vi "VA_ExtractImg32.vi"(1 "y":sgl, 2 "x":sgl, 3 "Image Src":T1) -> (0 "Image Dst Out":T1)   [LabVIEW 2009]
uses:
  <vilib>/vision/Image Controls.llb/IMAQ Image.ctl
  <vilib>/vision/NI_Vision_Development_Module.lvlib
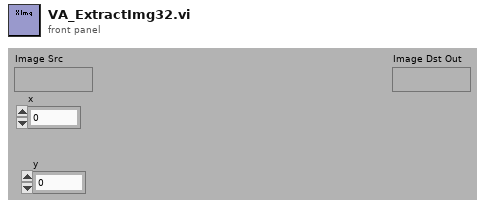
[diagram p1: front panel]
types:
  T1 = typedef "IMAQ Image.ctl" = refnum<image>
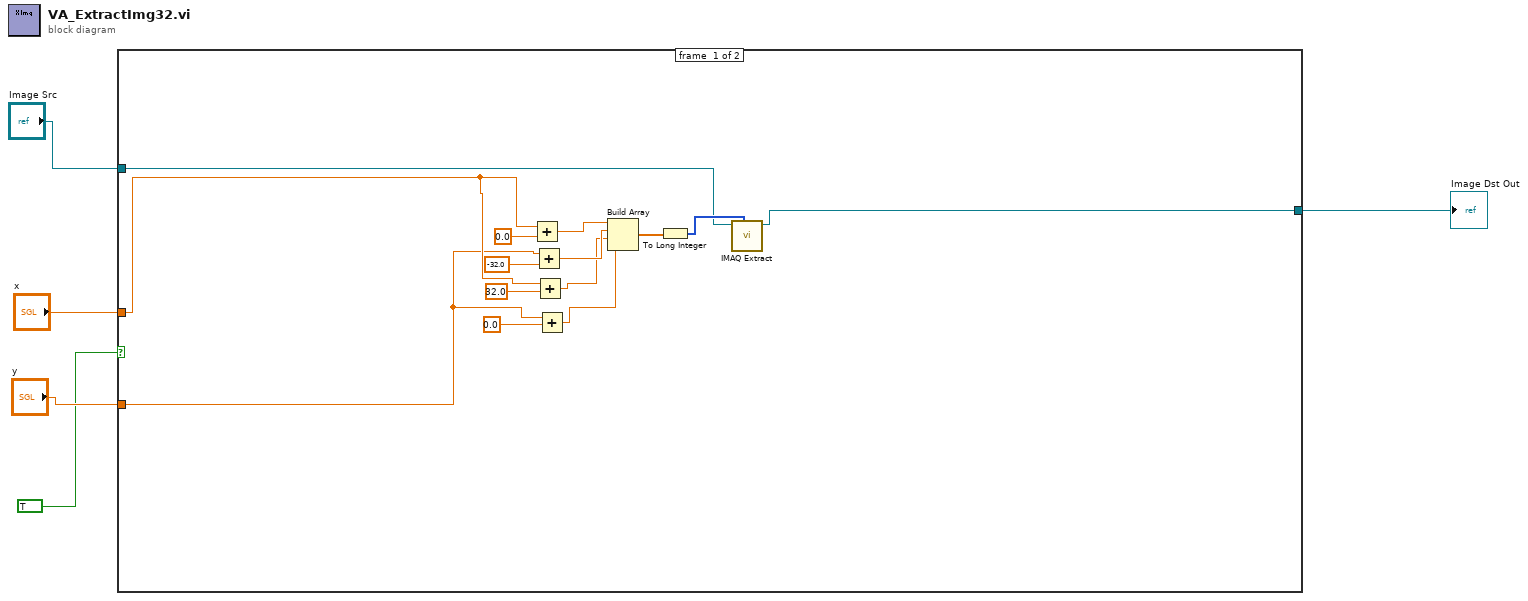
[diagram p0: block diagram]
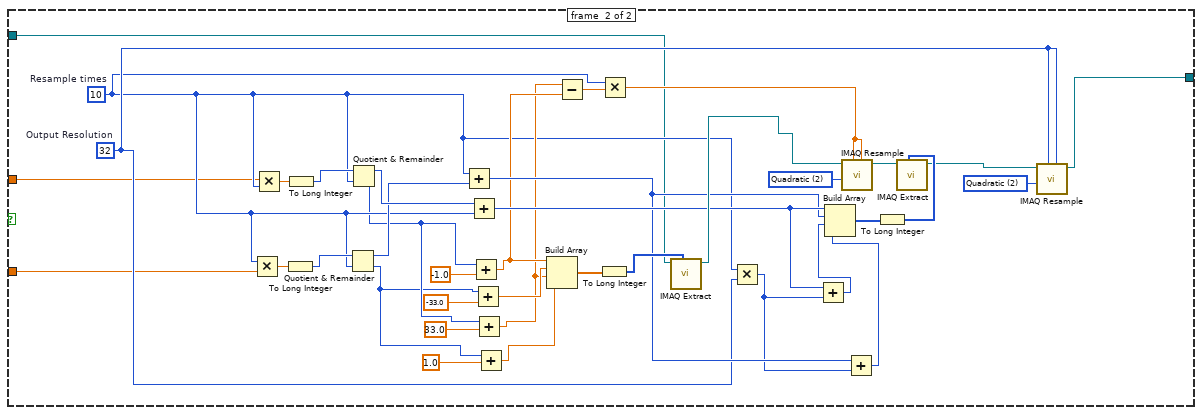
[diagram p2: hidden frame]
diagram:
  n1 = case shown="True" TRUE {
    tunnel: [w6 w34] -> w5
    tunnel: "Image Src" -> [w7 w22]
    tunnel: "x" -> [w9 w21]
    tunnel: "y" -> [w8 w20]
    frame #0 {
      n2 = Add(x=w9, y=sgl 0.0) -> (x+y=w11:sgl)
      n3 = Add(x=w8, y=sgl -32.0) -> (x+y=w19:sgl)
      n4 = Add(x=w9, y=sgl 32.0) -> (x+y=w10:sgl)
      n5 = Add(x=w8, y=sgl 0.0) -> (x+y=w14:sgl)
      n6 = Build Array(w11, w19, w10, w14) -> (w13:sgl[])
      n7 = To Long Integer(number=w13) -> (32bit integer=w12:i32[])
      n8 = call "IMAQ Extract"("Optional Rectangle"=w12, "Image Src"=w7) -> ("Image Dst Out"=w6:T1)  [unwired: 8 in, 1 out]
    }
    frame #1 {
      w27 = 32  # Output Resolution
      w36 = u32 2 items=["Zero Order", "Bi-Linear", "Quadratic", "Cubic Spline"] ("Interpolation Type")
      w45 = u32 2 items=["Zero Order", "Bi-Linear", "Quadratic", "Cubic Spline"] ("Interpolation Type")
      w26 = 10  # Resample times
      n9 = Multiply(x=w26, y=w20) -> (x*y=w49:sgl)
      n10 = Multiply(x=w21, y=w26) -> (x*y=w48:sgl)
      n11 = To Long Integer(number=w49) -> (32bit integer=w46:i32)
      n12 = To Long Integer(number=w48) -> (32bit integer=w47:i32)
      n13 = Quotient & Remainder(x=w46, y=w26) -> (x-y*floor(x/y)=w40:i32, floor(x/y)=w23:i32)
      n14 = Quotient & Remainder(x=w47, y=w26) -> (x-y*floor(x/y)=w42:i32, floor(x/y)=w24:i32)
      n15 = Add(x=w26, y=w40) -> (x+y=w32:i32)
      n16 = Add(x=w42, y=w26) -> (x+y=w33:i32)
      n17 = Add(x=w24, y=sgl -1.0) -> (x+y=w31:sgl)
      n18 = Add(x=w23, y=sgl -33.0) -> (x+y=w57:sgl)
      n19 = Add(x=w24, y=sgl 33.0) -> (x+y=w30:sgl)
      n20 = Add(x=w23, y=sgl 1.0) -> (x+y=w52:sgl)
      n21 = Build Array(w31, w57, w30, w52) -> (w51:sgl[])
      n22 = Subtract(x=w30, y=w31) -> (x-y=w29:sgl)
      n23 = To Long Integer(number=w51) -> (32bit integer=w50:i32[])
      n24 = Multiply(x=w26, y=w29) -> (x*y=w28:sgl)
      n25 = call "IMAQ Extract"("Optional Rectangle"=w50, "Image Src"=w22) -> ("Image Dst Out"=w44:T1)  [unwired: 8 in, 1 out]
      n26 = Multiply(x=w26, y=w27) -> (x*y=w25:i32)
      n27 = Add(x=w33, y=w25) -> (x+y=w41:i32)
      n28 = call "IMAQ Resample"("X Resolution"=w28, "Y Resolution"=w28, "Interpolation Type"=w45, "Image Src"=w44) -> ("Image Dst Out"=w37:T1)  [unwired: 6 in, 1 out]
      n29 = Add(x=w32, y=w25) -> (x+y=w39:i32)
      n30 = Build Array(w33, w32, w41, w39) -> (w43:i32[])
      n31 = To Long Integer(number=w43) -> (32bit integer=w38:i32[])
      n32 = call "IMAQ Extract"("Optional Rectangle"=w38, "Image Src"=w37) -> ("Image Dst Out"=w35:T1)  [unwired: 8 in, 1 out]
      n33 = call "IMAQ Resample"("X Resolution"=w27, "Y Resolution"=w27, "Interpolation Type"=w36, "Image Src"=w35) -> ("Image Dst Out"=w34:T1)  [unwired: 6 in, 1 out]
    }
  }
  "Image Dst Out" <- w5
